vi "ConfigTDC.vi"(6 "# Evts to Acquire":u16=1, 7 "Interrupt Level":u16=1, 8 "error in (no error)":errorcluster, 9 "FSR setting":u16=90 format="%.0x", 10 "handle":i32, 11 "VME Base Address":u32 format="%.0x") -> (0 "error out":errorcluster, 3 "handle out":i32)   [LabVIEW 2014]
uses:
  Program Files (x86)/CAEN/Comm/labview/CAENComm.lvlib
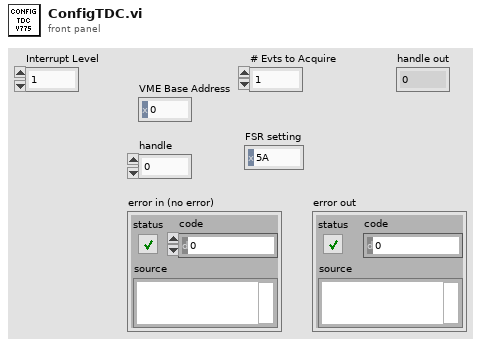
[diagram p1: front panel]
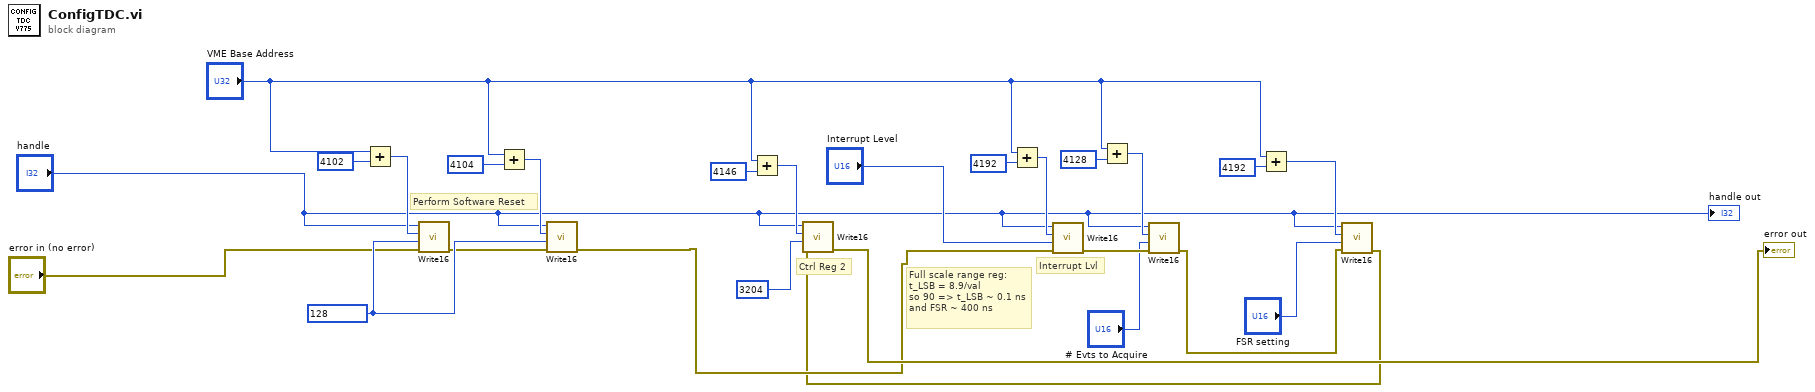
[diagram p0: block diagram]
diagram:
  w24 = u16 128 ("Data")
  # "Interrupt Lvl"
  # "Full scale range reg:\nt_LSB = 8.9/val\nso 90 => t_LSB ~ 0.1 ns\nand FSR ~ 400 ns"
  # "Ctrl Reg 2"
  # "Perform Software Reset"
  n1 = Add(x="VME Base Address", y=u32 4102) -> (x+y=w19:u32)
  n2 = call "Write16.vi"("error in (no error)"="error in (no error)", "Data"=w24, "Address"=w19, "handle"="handle") -> ("error out"=w21:errorcluster)  [unwired: 7 in]
  n3 = Add(x="VME Base Address", y=u32 4104) -> (x+y=w23:u32)
  n4 = call "Write16.vi"("error in (no error)"=w21, "Data"=w24, "Address"=w23, "handle"="handle") -> ("error out"=w3:errorcluster)  [unwired: 7 in]
  n5 = Add(x="VME Base Address", y=u32 4146) -> (x+y=w26:u32)
  n6 = Add(x="VME Base Address", y=u32 4192) -> (x+y=w15:u32)
  n7 = call "Write16.vi"("error in (no error)"=w3, "Data"="Interrupt Level", "Address"=w15, "handle"="handle") -> ("error out"=w13:errorcluster)  [unwired: 7 in]
  n8 = Add(x="VME Base Address", y=u32 4128) -> (x+y=w11:u32)
  n9 = call "Write16.vi"("error in (no error)"=w13, "Data"="# Evts to Acquire", "Address"=w11, "handle"="handle") -> ("error out"=w2:errorcluster)  [unwired: 7 in]
  n10 = Add(x="VME Base Address", y=u32 4192) -> (x+y=w8:u32)
  n11 = call "Write16.vi"("error in (no error)"=w2, "Data"="FSR setting", "Address"=w8, "handle"="handle") -> ("error out"=w1:errorcluster)  [unwired: 7 in]
  n12 = call "Write16.vi"("error in (no error)"=w1, "Data"=u16 3204, "Address"=w26, "handle"="handle") -> ("error out"=→"error out":errorcluster)  [unwired: 7 in]
  "handle out" <- "handle"
